vi "write test setp.vi"(0 "Write step":T1, 1 "Pass/Fail":bool, 2 "In value 1":string, 3 "In value 2":string, 4 "In value 3":string, 5 "In value 4":string, 6 "In value 5":string, 7 "In value 6":string, 8 "Test_1":bool=TRUE, 10 "Test_2":bool=TRUE, 12 "Test_3":bool=TRUE, 14 "Test_4":bool=TRUE, 16 "Test_5":bool=TRUE, 18 "Test_6":bool=TRUE) -> (20 "字符串 2":string)   [LabVIEW 2009]
uses:
  write step control.ctl
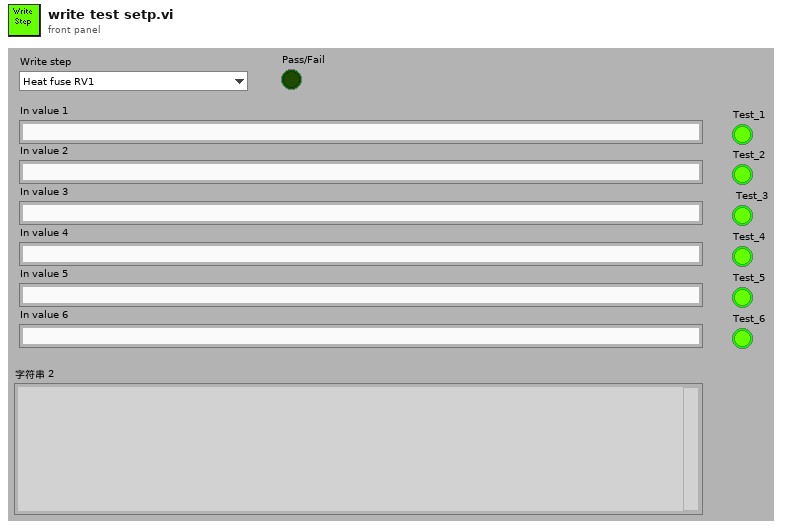
[diagram p1: front panel]
types:
  T1 = typedef "write step control.ctl" = enum16{"Heat fuse RV1", "Overriding diode D1", "Test firmware file upload", "Temperature sensor", "Real-time clock accuracy", "I2C Communication on Z1", "Light-emitting diode on Z2", "Battery warning/inhibit", "Reset by IC10", "External EEPROM", "RFID card detection and reading", "Production parameters in internal EEPROM", "Current consumption in sleep mode", "Application and database upload"}
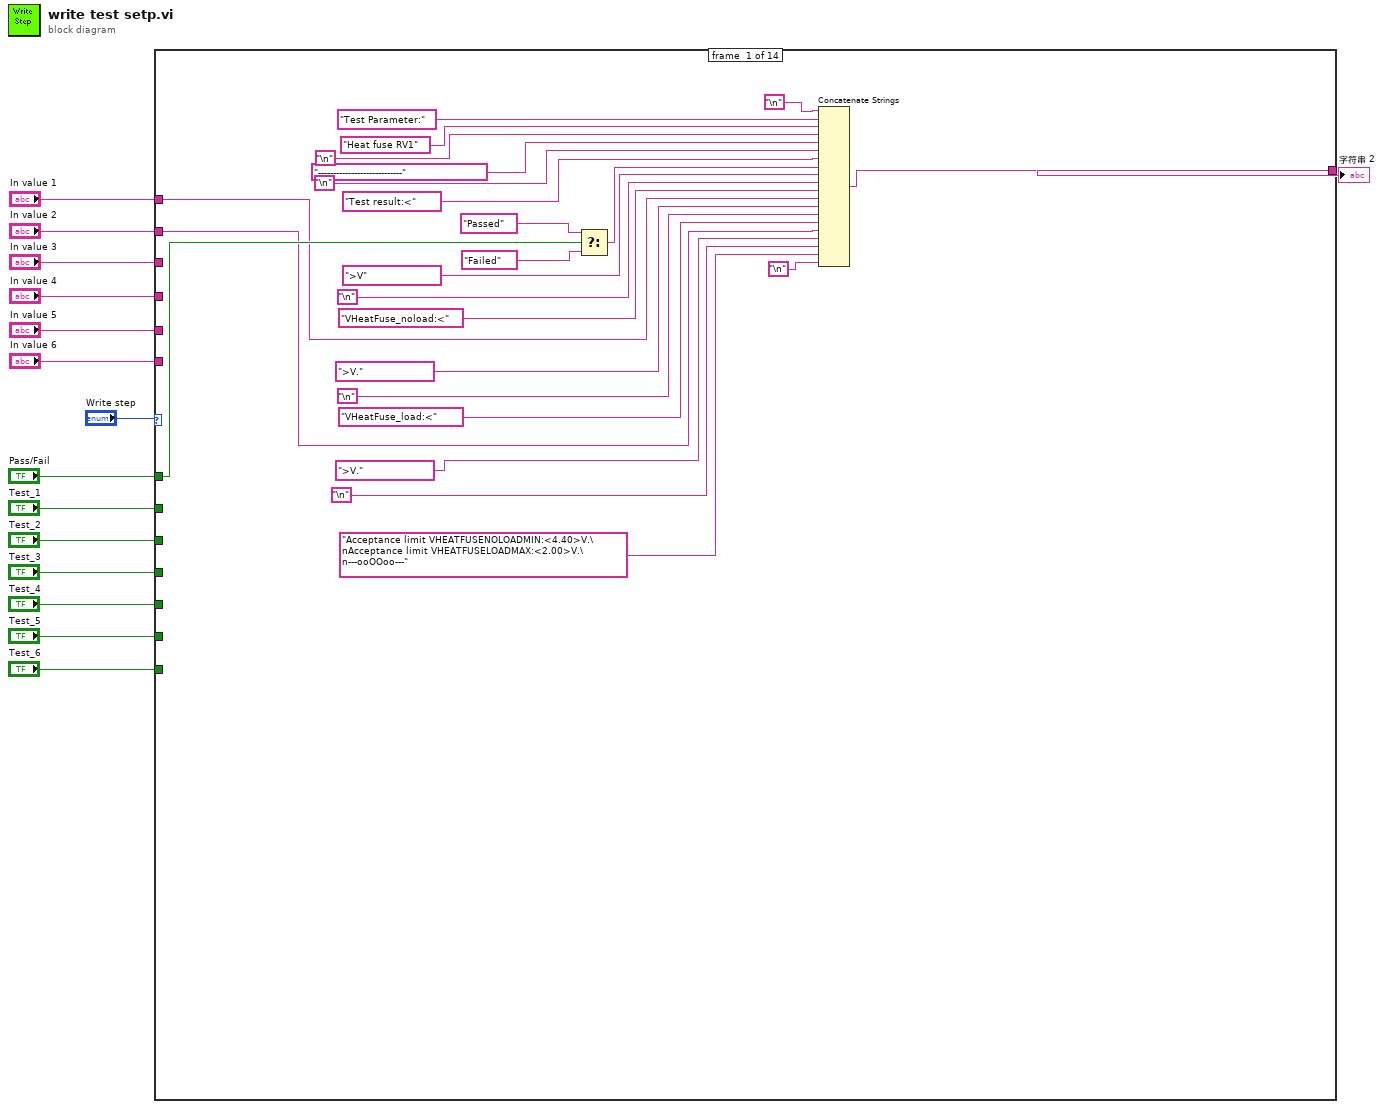
[diagram p0: block diagram]
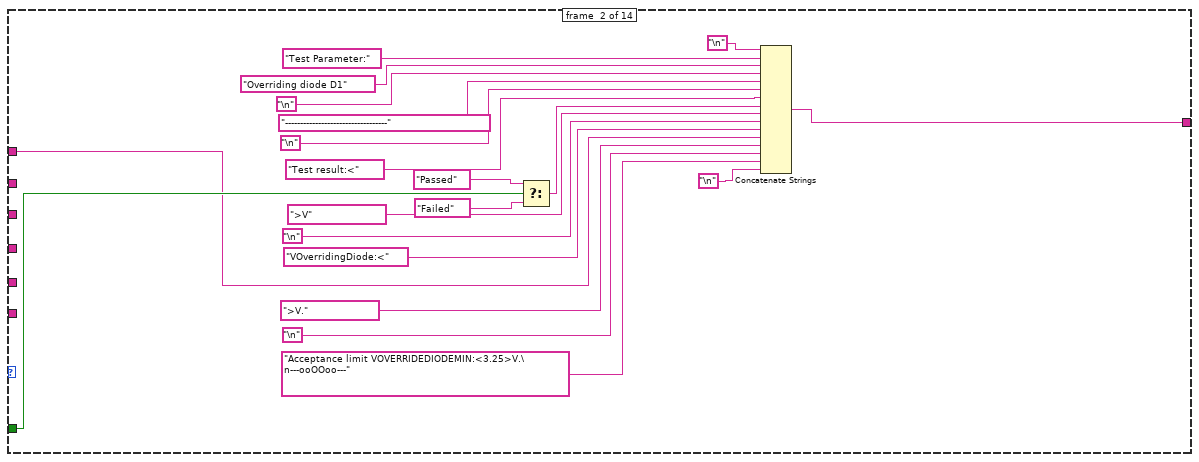
[diagram p2: hidden frame]
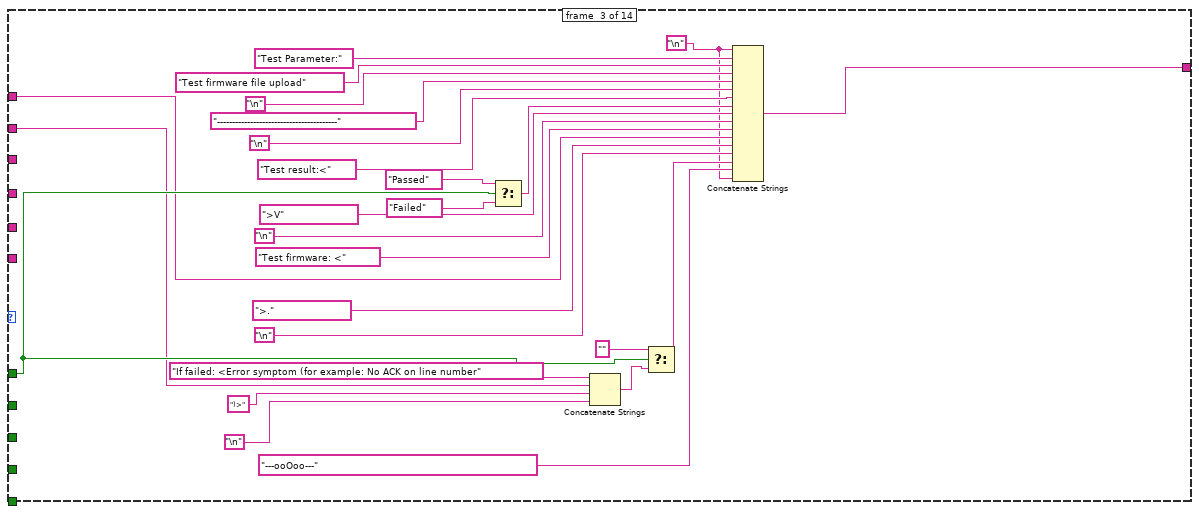
[diagram p3: hidden frame]
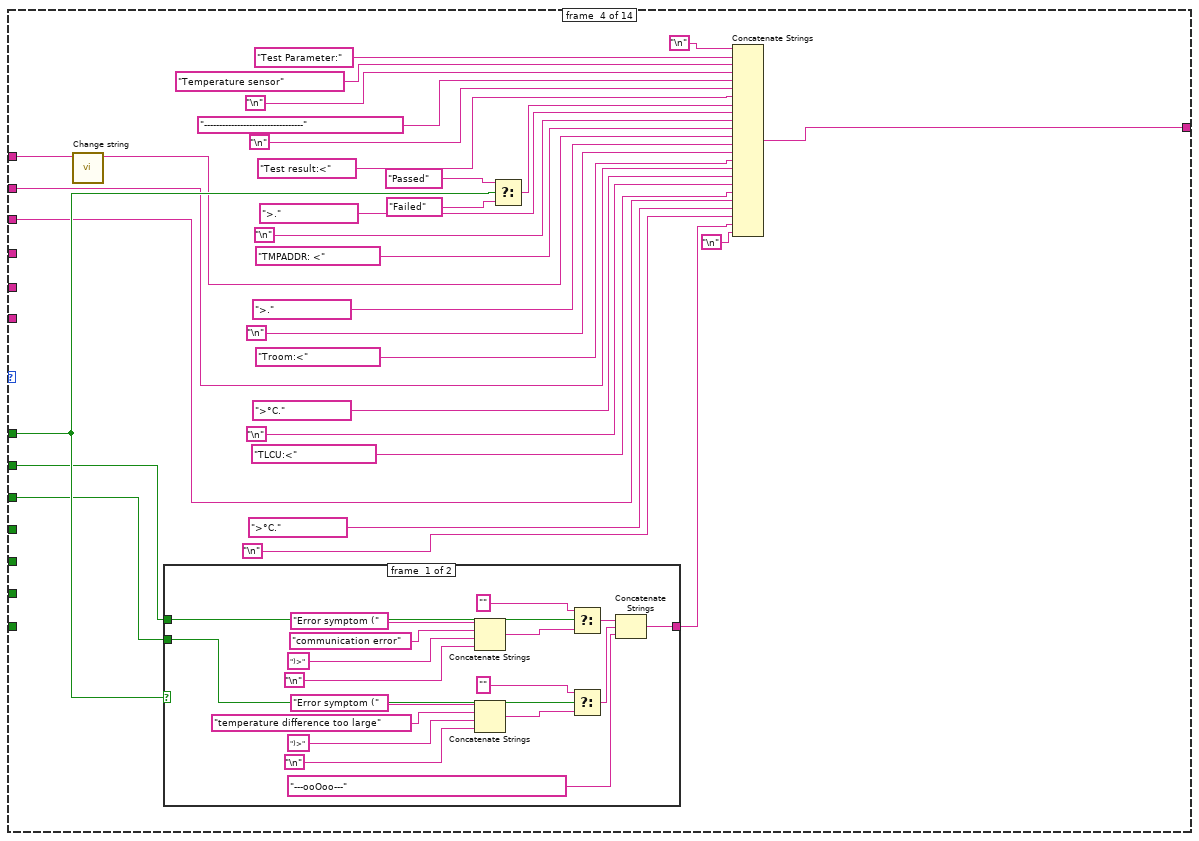
[diagram p4: hidden frame]
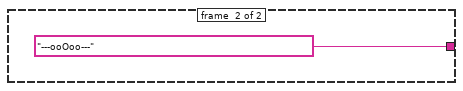
[diagram p5: hidden frame]
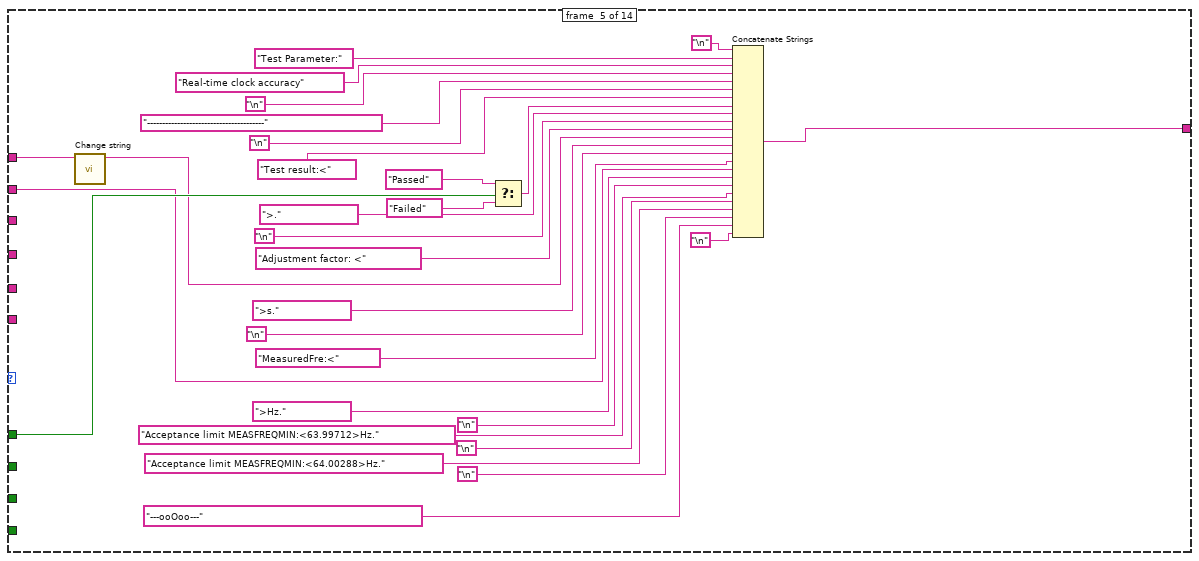
[diagram p6: hidden frame]
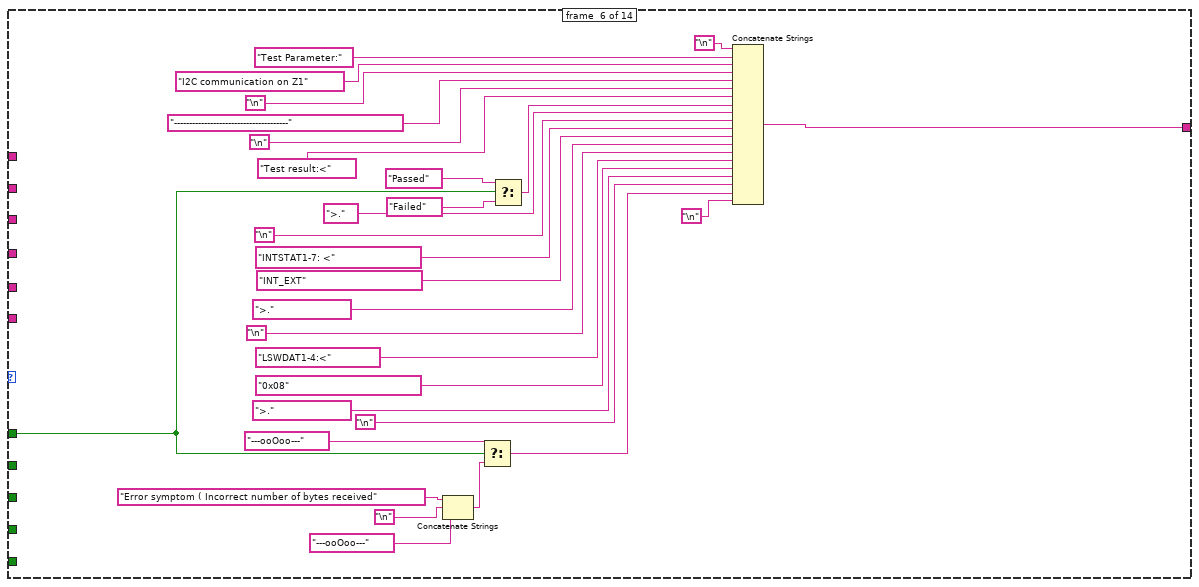
[diagram p7: hidden frame]
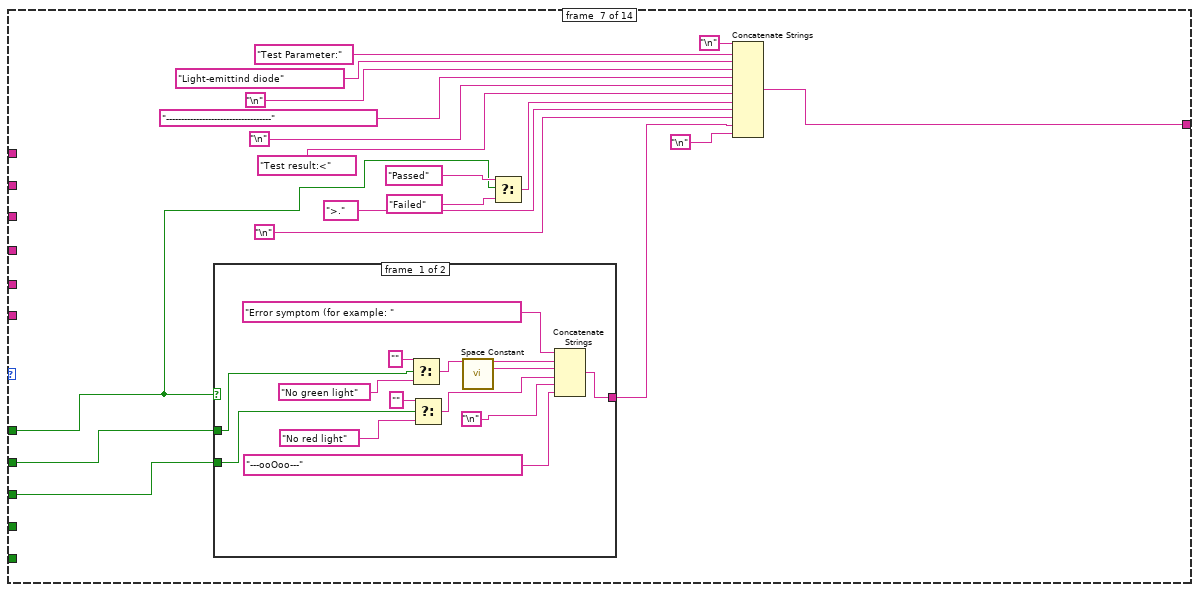
[diagram p8: hidden frame]
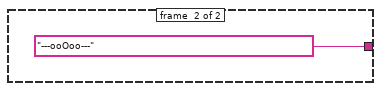
[diagram p9: hidden frame]
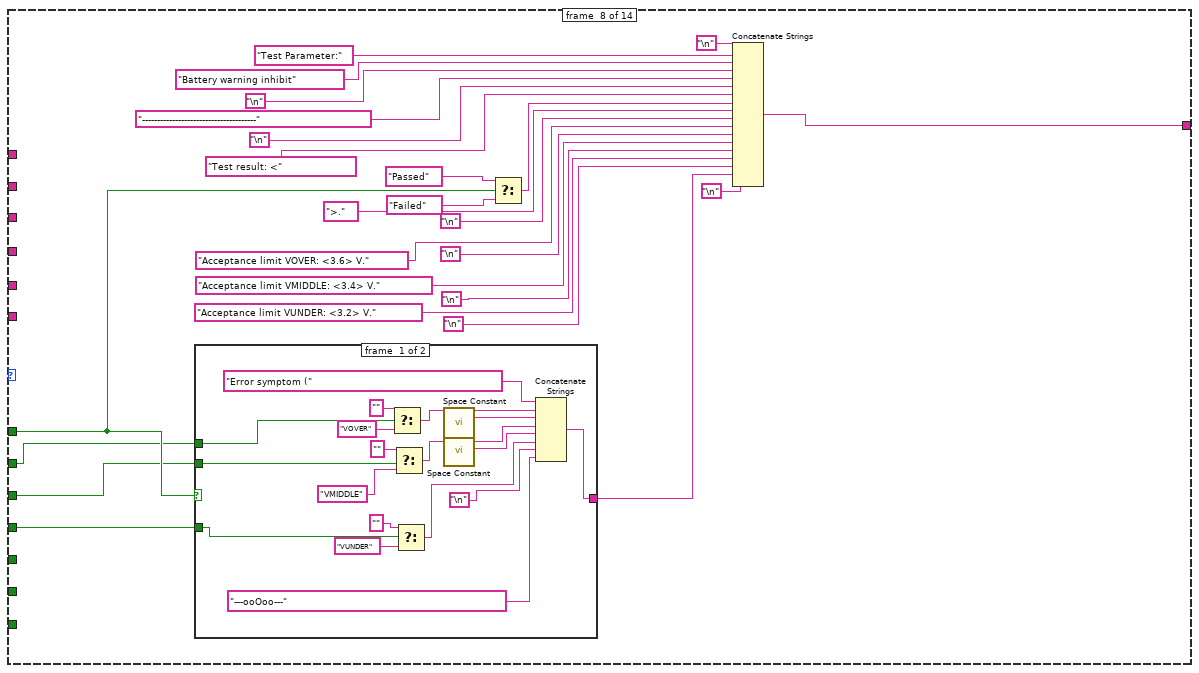
[diagram p10: hidden frame]
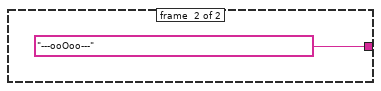
[diagram p11: hidden frame]
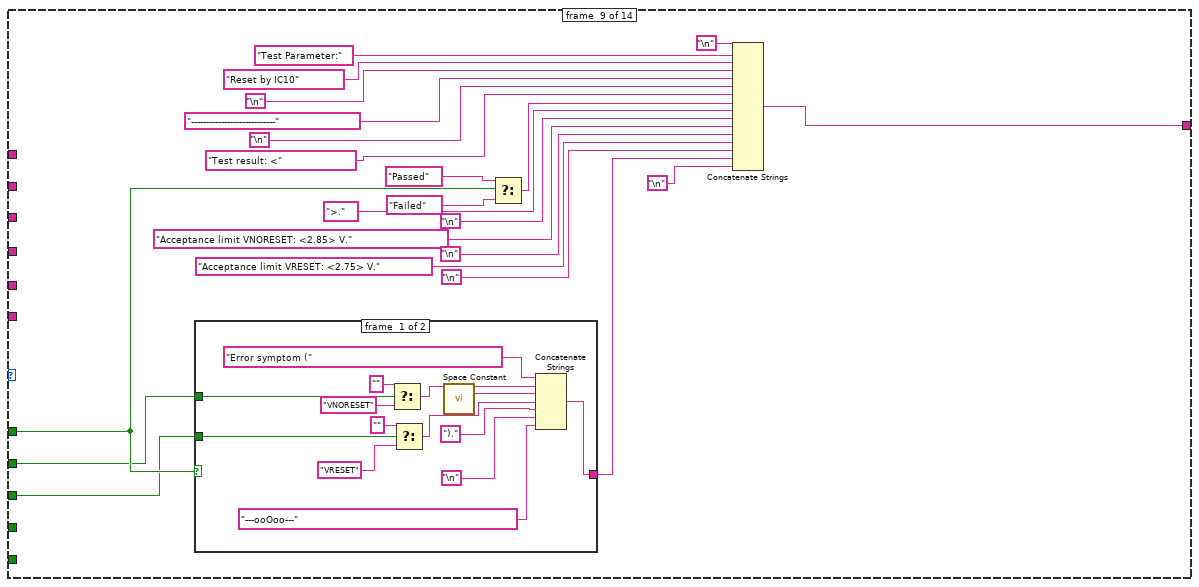
[diagram p12: hidden frame]
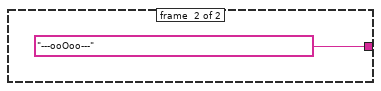
[diagram p13: hidden frame]
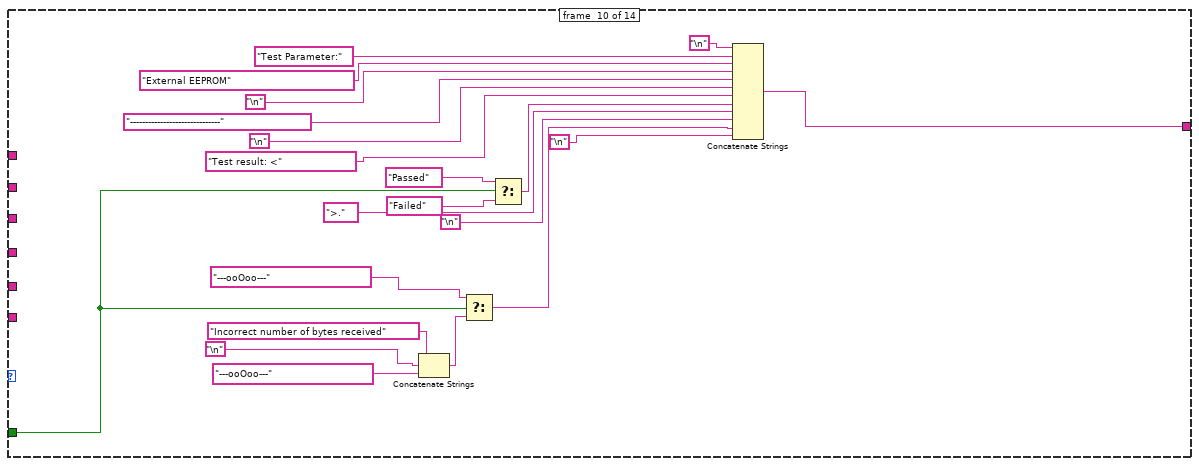
[diagram p14: hidden frame]
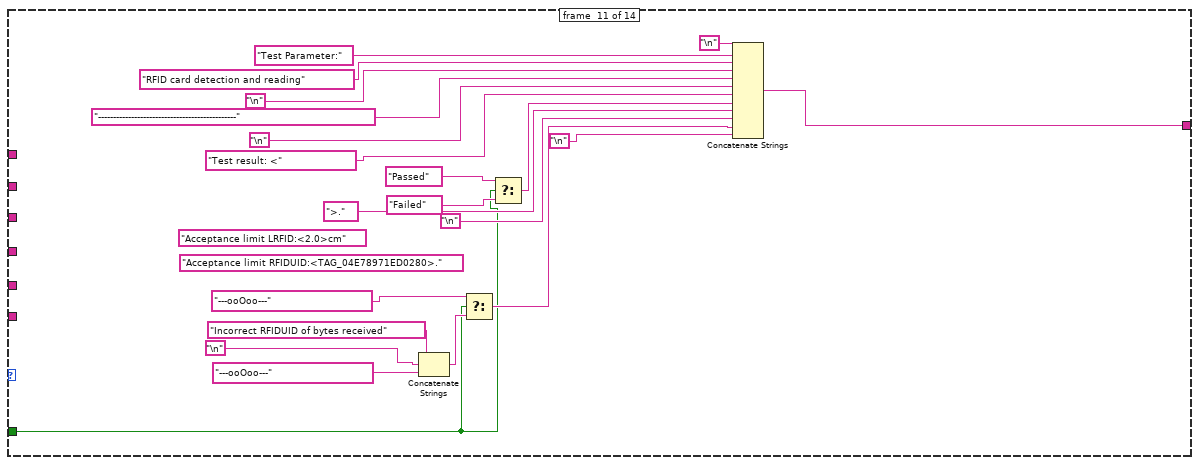
[diagram p15: hidden frame]
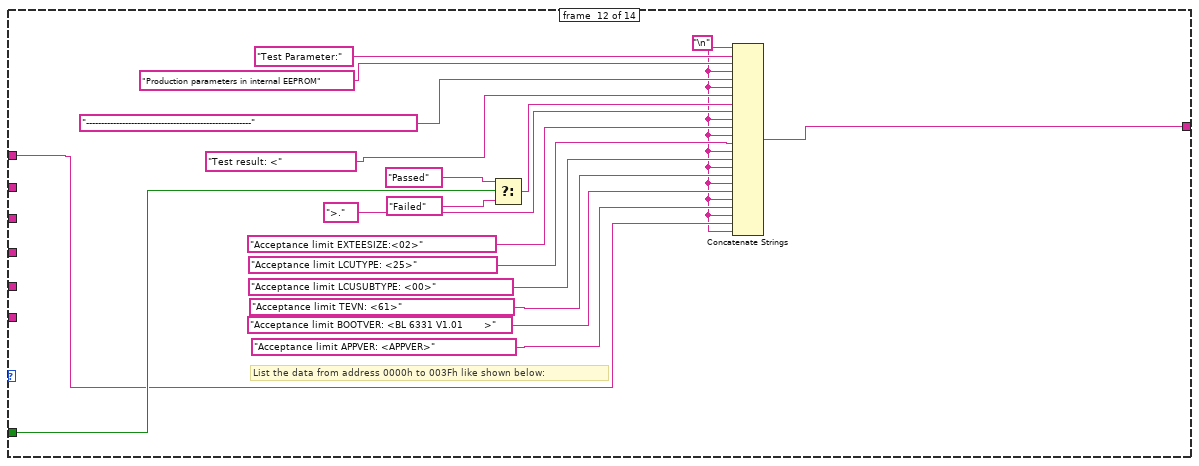
[diagram p16: hidden frame]
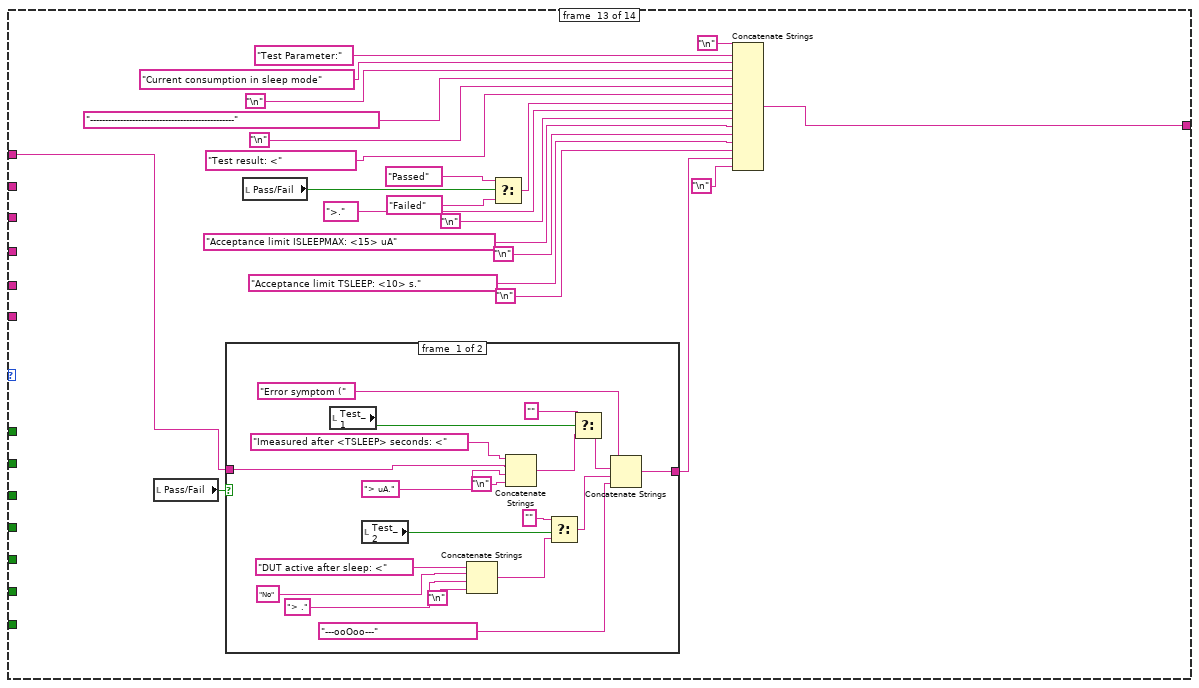
[diagram p17: hidden frame]
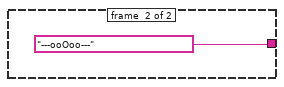
[diagram p18: hidden frame]
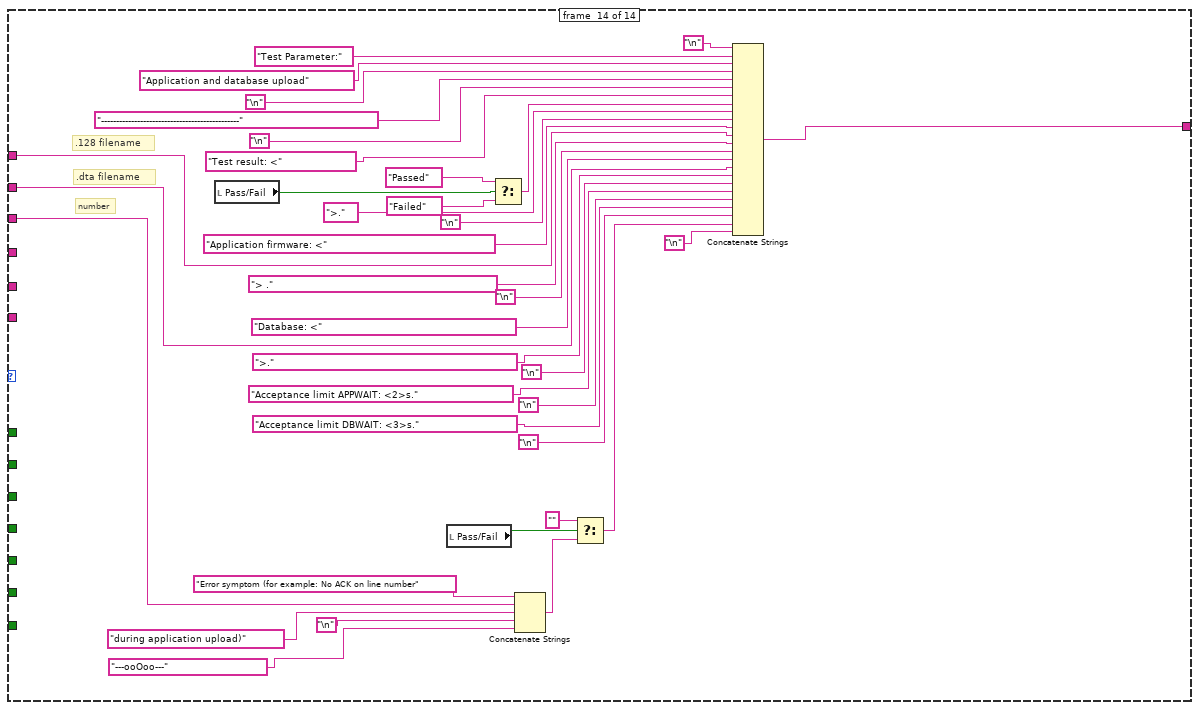
[diagram p19: hidden frame]
diagram:
  n1 = case shown="\"Application and database upload\"" "Write step" {
    tunnel: [w21 w56 w64 w102 w150 w179 w200 w239 w280 w316 w337 w358 w377 w433] -> w15
    tunnel: "Pass/Fail" -> [w18 w43 w63 w93 w140 w174 w195 w229 w273 w308 w329 w351 _ _]
    tunnel: "Test_1" -> [_ _ _ w92 _ _ w197 w228 w272 _ _ _ _ _]
    tunnel: "Test_2" -> [_ _ _ w91 _ _ w196 w227 w271 _ _ _ _ _]
    tunnel: "Test_3" -> [_ _ _ _ _ _ _ w230 _ _ _ _ _ _]
    tunnel: "Test_4" -> [_ _ _ _ _ _ _ _ _ _ _ _ _ _]
    tunnel: "Test_5" -> [_ _ _ _ _ _ _ _ _ _ _ _ _ _]
    tunnel: "Test_6" -> [_ _ _ _ _ _ _ _ _ _ _ _ _ _]
    tunnel: "In value 1" -> [w17 w42 w62 w87 w137 _ _ _ _ _ _ w350 w368 w411]
    tunnel: "In value 2" -> [w16 _ w61 w90 w139 _ _ _ _ _ _ _ _ w410]
    tunnel: "In value 3" -> [_ _ _ w89 _ _ _ _ _ _ _ _ _ w409]
    tunnel: "In value 4" -> [_ _ _ _ _ _ _ _ _ _ _ _ _ _]
    tunnel: "In value 5" -> [_ _ _ _ _ _ _ _ _ _ _ _ _ _]
    tunnel: "In value 6" -> [_ _ _ _ _ _ _ _ _ _ _ _ _ _]
    frame #0 {
      n2 = Select(t="Passed", s=w18, f="Failed") -> (s? t:f=w31:string)
      n3 = Concatenate Strings("\n", "Test Parameter:", "Heat fuse RV1", "\n", "----------------------------", "\n", "Test result:<", w31, ">V", "\n", "VHeatFuse_noload:<", w17, ">V.", "\n", "VHeatFuse_load:<", w16, ">V.", "\n", "Acceptance limit VHEATFUSENOLOADMIN:<4.40>V.\nAcceptance limit VHEATFUSELOADMAX:<2.00>V.\n---ooOOoo---", "\n") -> (w21:string)
    }
    frame #1 {
      n4 = Select(t="Passed", s=w43, f="Failed") -> (s? t:f=w50:string)
      n5 = Concatenate Strings("\n", "Test Parameter:", "Overriding diode D1", "\n", "----------------------------------", "\n", "Test result:<", w50, ">V", "\n", "VOverridingDiode:<", w42, ">V.", "\n", "Acceptance limit VOVERRIDEDIODEMIN:<3.25>V.\n---ooOOoo---", "\n") -> (w56:string)
    }
    frame #2 {
      w60 = "\n"
      n6 = Select(t="Passed", s=w63, f="Failed") -> (s? t:f=w77:string)
      n7 = Concatenate Strings("If failed: <Error symptom (for example: No ACK on line number" ("字符串"), w61, ")>" ("字符串"), "\n") -> (w70:string)
      n8 = Select(t="", s=w63, f=w70) -> (s? t:f=w67:string)
      n9 = Concatenate Strings(w60, "Test Parameter:", "Test firmware file upload", "\n", "----------------------------------------", "\n", "Test result:<", w77, ">V", "\n", "Test firmware: <", w62, ">.", "\n", w67, "---ooOoo---", w60) -> (w64:string)
    }
    frame #3 {
      n10 = call "Change string.vi"("string"=w87) -> ("String"=w86:string)  [unwired: 10 out]
      n11 = case shown="False" w93 {
        tunnel: [w117 "---ooOoo---"] -> w95
        tunnel: w91 -> [w122 _]
        tunnel: w92 -> [w121 _]
        frame #0 {
          n12 = Concatenate Strings("Error symptom (" ("字符串"), "communication error" ("字符串"), ")>" ("字符串"), "\n") -> (w130:string)
          n13 = Concatenate Strings("Error symptom (" ("字符串"), "temperature difference too large" ("字符串"), ")>" ("字符串"), "\n") -> (w127:string)
          n14 = Select(t="", s=w121, f=w130) -> (s? t:f=w120:string)
          n15 = Select(t="", s=w122, f=w127) -> (s? t:f=w119:string)
          n16 = Concatenate Strings(w120, w119, "---ooOoo---") -> (w117:string)
        }
        frame #1 {
        }
      }
      n17 = Select(t="Passed", s=w93, f="Failed") -> (s? t:f=w108:string)
      n18 = Concatenate Strings("\n", "Test Parameter:", "Temperature sensor", "\n", "---------------------------------", "\n", "Test result:<", w108, ">.", "\n", "TMPADDR: <", w86, ">.", "\n", "Troom:<", w90, ">°C.", "\n", "TLCU:<", w89, ">°C.", "\n", w95, "\n") -> (w102:string)
    }
    frame #4 {
      n19 = call "Change string.vi"("string"=w137) -> ("String"=w136:string)  [unwired: 10 out]
      n20 = Select(t="Passed", s=w140, f="Failed") -> (s? t:f=w156:string)
      n21 = Concatenate Strings("\n", "Test Parameter:", "Real-time clock accuracy", "\n", "---------------------------------------", "\n", "Test result:<", w156, ">.", "\n", "Adjustment factor: <", w136, ">s.", "\n", "MeasuredFre:<", w139, ">Hz.", "\n", "Acceptance limit MEASFREQMIN:<63.99712>Hz.", "\n", "Acceptance limit MEASFREQMIN:<64.00288>Hz.", "\n", "---ooOoo---", "\n") -> (w150:string)
    }
    frame #5 {
      n22 = Concatenate Strings("Error symptom ( Incorrect number of bytes received", "\n", "---ooOoo---") -> (w167:string)
      n23 = Select(t="---ooOoo---", s=w174, f=w167) -> (s? t:f=w175:string)
      n24 = Select(t="Passed", s=w174, f="Failed") -> (s? t:f=w185:string)
      n25 = Concatenate Strings("\n", "Test Parameter:", "I2C communication on Z1", "\n", "--------------------------------------", "\n", "Test result:<", w185, ">.", "\n", "INTSTAT1-7: <", "INT_EXT", ">.", "\n", "LSWDAT1-4:<", "0x08", ">.", "\n", w175, "\n") -> (w179:string)
    }
    frame #6 {
      n26 = case shown="True" w195 {
        tunnel: [w218 "---ooOoo---"] -> w199
        tunnel: w197 -> [w213 _]
        tunnel: w196 -> [w212 _]
        frame #0 {
          n27 = Select(t="", s=w213, f="No green light") -> (s? t:f=w219:string)
          n28 = Select(t="", s=w212, f="No red light") -> (s? t:f=w217:string)
          n29 = call <vilib>:"Space Constant.vi"() -> ("String"=w215:string)
          n30 = Concatenate Strings("Error symptom (for example: ", w219, w215, w217, "\n", "---ooOoo---") -> (w218:string)
        }
        frame #1 {
        }
      }
      n31 = Select(t="Passed", s=w195, f="Failed") -> (s? t:f=w203:string)
      n32 = Concatenate Strings("\n", "Test Parameter:", "Light-emittind diode", "\n", "-----------------------------------", "\n", "Test result:<", w203, ">.", "\n", w199, "\n") -> (w200:string)
    }
    frame #7 {
      n33 = case shown="False" w229 {
        tunnel: [w263 "---ooOoo---"] -> w232
        tunnel: w228 -> [w253 _]
        tunnel: w227 -> [w252 _]
        tunnel: w230 -> [w251 _]
        frame #0 {
          n34 = Select(t="", s=w253, f="VOVER") -> (s? t:f=w264:string)
          n35 = Select(t="", s=w252, f="VMIDDLE") -> (s? t:f=w262:string)
          n36 = Select(t="", s=w251, f="VUNDER") -> (s? t:f=w256:string)
          n37 = call <vilib>:"Space Constant.vi"() -> ("String"=w261:string)
          n38 = call <vilib>:"Space Constant.vi"() -> ("String"=w257:string)
          n39 = Concatenate Strings("Error symptom (", w264, w261, w262, w257, w256, "\n", "---ooOoo---") -> (w263:string)
        }
        frame #1 {
        }
      }
      n40 = Select(t="Passed", s=w229, f="Failed") -> (s? t:f=w242:string)
      n41 = Concatenate Strings("\n", "Test Parameter:", "Battery warning inhibit", "\n", "--------------------------------------", "\n", "Test result: <", w242, ">.", "\n", "Acceptance limit VOVER: <3.6> V.", "\n", "Acceptance limit VMIDDLE: <3.4> V.", "\n", "Acceptance limit VUNDER: <3.2> V.", "\n", w232, "\n") -> (w239:string)
    }
    frame #8 {
      n42 = case shown="False" w273 {
        tunnel: [w300 "---ooOoo---"] -> w275
        tunnel: w272 -> [w293 _]
        tunnel: w271 -> [w292 _]
        frame #0 {
          n43 = Select(t="", s=w293, f="VNORESET") -> (s? t:f=w301:string)
          n44 = Select(t="", s=w292, f="VRESET") -> (s? t:f=w299:string)
          n45 = call <vilib>:"Space Constant.vi"() -> ("String"=w298:string)
          n46 = Concatenate Strings("Error symptom (", w301, w298, w299, ").", "\n", "---ooOoo---") -> (w300:string)
        }
        frame #1 {
        }
      }
      n47 = Select(t="Passed", s=w273, f="Failed") -> (s? t:f=w283:string)
      n48 = Concatenate Strings("\n", "Test Parameter:", "Reset by IC10", "\n", "----------------------------", "\n", "Test result: <", w283, ">.", "\n", "Acceptance limit VNORESET: <2.85> V.", "\n", "Acceptance limit VRESET: <2.75> V.", "\n", w275, "\n") -> (w280:string)
    }
    frame #9 {
      n49 = Concatenate Strings("Incorrect number of bytes received", "\n", "---ooOoo---") -> (w312:string)
      n50 = Select(t="---ooOoo---", s=w308, f=w312) -> (s? t:f=w315:string)
      n51 = Select(t="Passed", s=w308, f="Failed") -> (s? t:f=w319:string)
      n52 = Concatenate Strings("\n", "Test Parameter:", "External EEPROM", "\n", "------------------------------", "\n", "Test result: <", w319, ">.", "\n", w315, "\n") -> (w316:string)
    }
    frame #10 {
      (unwired) "Acceptance limit RFIDUID:<TAG_04E78971ED0280>."
      (unwired) "Acceptance limit LRFID:<2.0>cm"
      n53 = Concatenate Strings("Incorrect RFIDUID of bytes received", "\n", "---ooOoo---") -> (w333:string)
      n54 = Select(t="---ooOoo---", s=w329, f=w333) -> (s? t:f=w336:string)
      n55 = Select(t="Passed", s=w329, f="Failed") -> (s? t:f=w340:string)
      n56 = Concatenate Strings("\n", "Test Parameter:", "RFID card detection and reading", "\n", "----------------------------------------------", "\n", "Test result: <", w340, ">.", "\n", w336, "\n") -> (w337:string)
    }
    frame #11 {
      w349 = "\n"
      # "List the data from address 0000h to 003Fh like shown below:"
      n57 = Select(t="Passed", s=w351, f="Failed") -> (s? t:f=w360:string)
      n58 = Concatenate Strings(w349, "Test Parameter:", "Production parameters in internal EEPROM", w349, "-------------------------------------------------------", w349, "Test result: <", w360, ">.", w349, "Acceptance limit EXTEESIZE:<02>", w349, "Acceptance limit LCUTYPE: <25>", w349, "Acceptance limit LCUSUBTYPE: <00>", w349, "Acceptance limit TEVN: <61>", w349, "Acceptance limit BOOTVER: <BL 6331 V1.01       >", w349, "Acceptance limit APPVER: <APPVER>", w349, w350, w349) -> (w358:string)
    }
    frame #12 {
      n59 = local read "Pass/Fail"() -> (w370:bool)
      n60 = case shown="False" w370 {
        tunnel: [w393 "---ooOoo---"] -> w372
        tunnel: w368 -> [w389 _]
        frame #0 {
          n61 = local read "Test_1"() -> (w391:bool)
          n62 = local read "Test_2"() -> (w390:bool)
          n63 = Concatenate Strings("DUT active after sleep: <", "No", "> .", "\n") -> (w398:string)
          n64 = Concatenate Strings("Imeasured after <TSLEEP> seconds: <", w389, "> uA.", "\n") -> (w399:string)
          n65 = Select(t="", s=w390, f=w398) -> (s? t:f=w396:string)
          n66 = Select(t="", s=w391, f=w399) -> (s? t:f=w397:string)
          n67 = Concatenate Strings("Error symptom (", w397, w396, "---ooOoo---") -> (w393:string)
        }
        frame #1 {
        }
      }
      n68 = local read "Pass/Fail"() -> (w369:bool)
      n69 = Select(t="Passed", s=w369, f="Failed") -> (s? t:f=w380:string)
      n70 = Concatenate Strings("\n", "Test Parameter:", "Current consumption in sleep mode", "\n", "------------------------------------------------", "\n", "Test result: <", w380, ">.", "\n", "Acceptance limit ISLEEPMAX: <15> uA", "\n", "Acceptance limit TSLEEP: <10> s.", "\n", w372, "\n") -> (w377:string)
    }
    frame #13 {
      # "number"
      # ".dta filename"
      # ".128 filename"
      n71 = local read "Pass/Fail"() -> (w413:bool)
      n72 = local read "Pass/Fail"() -> (w412:bool)
      n73 = Select(t="Passed", s=w413, f="Failed") -> (s? t:f=w436:string)
      n74 = Concatenate Strings("Error symptom (for example: No ACK on line number", w409, "during application upload)", "\n", "---ooOoo---") -> (w422:string)
      n75 = Select(t="", s=w412, f=w422) -> (s? t:f=w416:string)
      n76 = Concatenate Strings("\n", "Test Parameter:", "Application and database upload", "\n", "----------------------------------------------", "\n", "Test result: <", w436, ">.", "\n", "Application firmware: <", w411, "> .", "\n", "Database: <", w410, ">.", "\n", "Acceptance limit APPWAIT: <2>s.", "\n", "Acceptance limit DBWAIT: <3>s.", "\n", w416, "\n") -> (w433:string)
    }
  }
  "字符串 2" <- w15
